vi "validate.vi"(8 "error in":errorcluster, 11 "Shared Memory configuration in":refnum<class "Shared Memory configuration.lvclass">) -> (0 "error out":errorcluster, 3 "Shared Memory configuration out":refnum<class "Shared Memory configuration.lvclass">)   [LabVIEW 2013, in "Shared Memory configuration.lvclass"]
doc: "This function performs validation of the configuration. This function should be safe to call at any point and should not rely on anything in the runtime environment."
uses:
  Shared Memory configuration.lvclass
  <vilib>/NI/Tag Bus Module Framework/module configuration/TBM module configuration.lvclass
  Shared Memory configuration.lvclass/Shared Memory configuration.ctl
  <vilib>/NI/Tag Bus/tag/tag descriptor.lvclass/tag descriptor.ctl
  <vilib>/NI/Tag Bus Module Framework/channel/TBM channel.lvclass/TBM channel.ctl
  <vilib>/NI/Tag Bus/tag/read tag name.vi
  <vilib>/NI/Tag Bus/tag/read data type.vi
  <vilib>/NI/Tag Bus Module Framework/channel/Read channel classification.vi
  <vilib>/NI/Tag Bus Module Framework/channel/TBM channel.lvclass
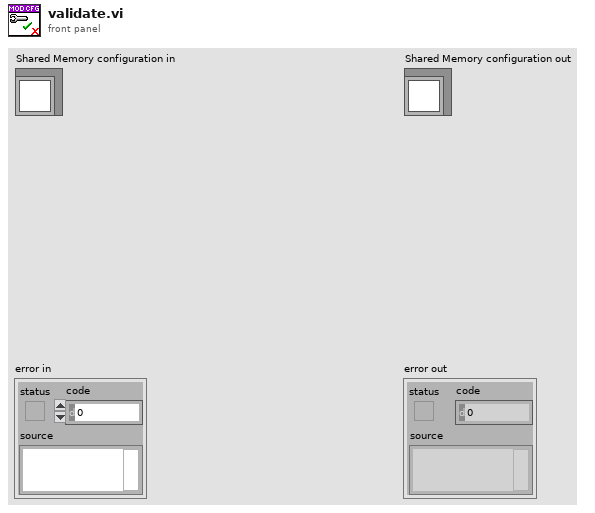
[diagram p1: front panel]
types:
  T1 = typedef "TBM channel.lvclass/channel classification.ctl" = enum16{"input data", "output data", "processing parameter", "processing result"}
  T2 = typedef "tag bus.lvlib/tag descriptor.lvclass/Data Type.ctl" = enum16{"Double", "Single", "I64", "I32", "I16", "I8", "U64", "U32", "U16", "U8", "Boolean", "String", "Array of Double", "Array of Single", "Array of I64", "Array of I32", "Array of I16", "Array of I8", "Array of U64", "Array of U32", "Array of U16", "Array of U8", "Array of Boolean", "Array of String"}
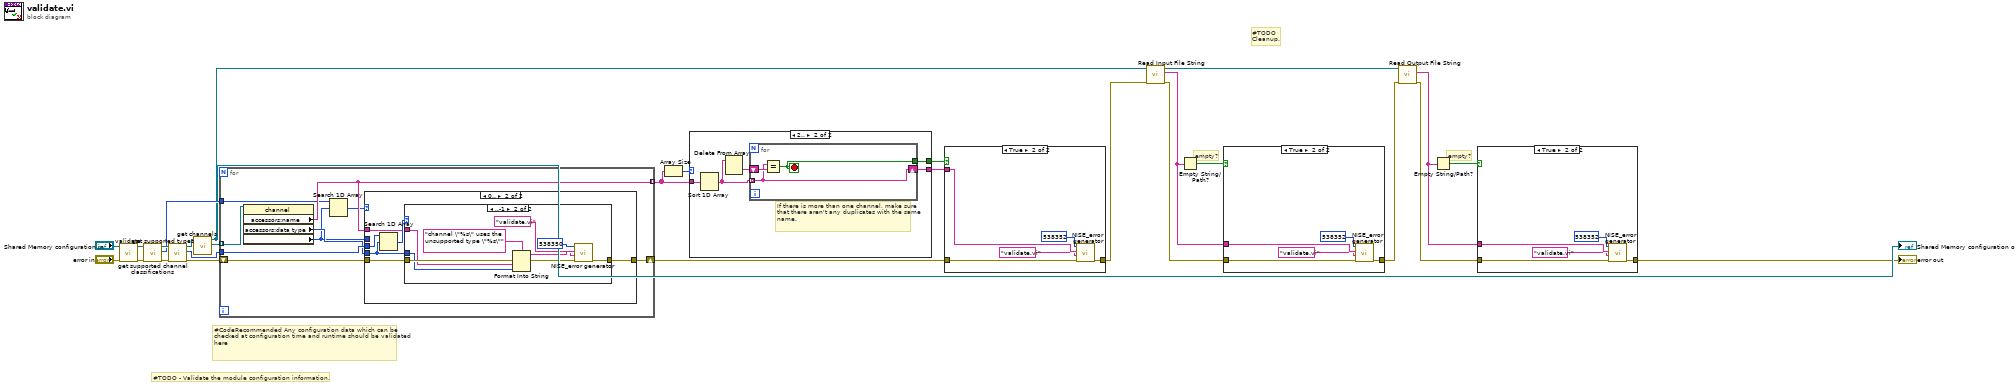
[diagram p0: block diagram]
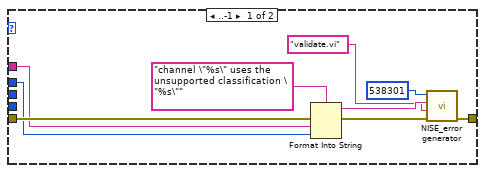
[diagram p6: hidden frame]
diagram:
  # "#TODO\nCleanup."
  # "empty?"
  # "empty?"
  # "#TODO - Validate the module configuration information."
  # "#CodeRecommended Any configuration data which can be checked at configuration time and runtime should be validated here"
  n1 = call-parent "validate.vi"("error in"="error in", "configuration in"="Shared Memory configuration in") -> ("error out"=w27:errorcluster, "configuration out"=w18:refnum<class "Shared Memory configuration.lvclass">)  [unwired: 8 in]
  n2 = call-dynamic "get supported channel classifications.vi"("error in"=w27, "module configuration in"=w18) -> ("error out"=w19:errorcluster, "supported classes"=w16:T1[], "module configuration out"=w17:refnum<class "Shared Memory configuration.lvclass">)  [unwired: 7 in]
  n3 = call-dynamic "get supported types.vi"("error in"=w19, "Shared Memory configuration in"=w17) -> ("error out"=w23:errorcluster, "supported types"=w24:T2[], "Shared Memory configuration out"=w26:refnum<class "Shared Memory configuration.lvclass">)  [unwired: 7 in]
  n4 = call-dynamic "get channels.vi"("Shared Memory configuration in"=w26) -> ("channels"=w25:refnum<class "TBM channel.lvclass">[], "Shared Memory configuration out"=w5:refnum<class "Shared Memory configuration.lvclass">)  [unwired: 9 in]
  "Shared Memory configuration out" <- w5
  n5 = for {
    tunnel: w25 -> [w36] mode=indexing
    tunnel: w24 -> [w35]
    shift-right: [w33] -> w14
    shift-left: w23 -> [w34]
    tunnel: [w31] -> w21 mode=indexing
    tunnel: w16 -> [w30]
    n6 = property class="channel"(reference=w36) -> ("accessors:name"=w31:string, "accessors:data type"=w32:T2, "data access:channel classification"=w28:T1)  [unwired: 1 in, 2 out]
    n7 = Search 1D Array(1D array=w30, element=w28) -> (index of element=w29:i32)  [unwired: 1 in]
    n8 = case shown="0.." w29 {
      tunnel: w35 -> [_ w51]
      tunnel: w34 -> [w41 w49]
      tunnel: [w40 w48] -> w33
      tunnel: w32 -> [_ w47]
      tunnel: w31 -> [w37 w46]
      tunnel: w28 -> [w38 _]
      frame ..-1 {
        n9 = Format Into String(format string="channel \"%s\" uses the unsupported classification \"%s\"", error in=w41, w37, w38) -> (resulting string=w43:string, error out=w44:errorcluster)  [unwired: 1 in]
        n10 = call <vilib>:"NISE_error generator.vi"("error in"=w44, "source"="validate.vi" ("format string"), "append error message"=w43, "error code (0)"=538301) -> ("error out"=w40:errorcluster)  [unwired: 5 in]
      }
      frame 0.. {
        n11 = Search 1D Array(1D array=w51, element=w47) -> (index of element=w50:i32)  [unwired: 1 in]
        n12 = case shown="..-1" w50 {
          tunnel: w49 -> [w52 w56]
          tunnel: [w52 w55] -> w48
          tunnel: w47 -> [_ w54]
          tunnel: w46 -> [_ w53]
          frame 0.. {
          }
          frame ..-1 {
            n13 = Format Into String(format string="channel \"%s\" uses the unsupported type \"%s\"", error in=w56, w53, w54) -> (resulting string=w59:string, error out=w60:errorcluster)  [unwired: 1 in]
            n14 = call <vilib>:"NISE_error generator.vi"("error in"=w60, "source"="validate.vi" ("format string"), "append error message"=w59, "error code (0)"=538350) -> ("error out"=w55:errorcluster)  [unwired: 5 in]
          }
        }
      }
    }
  }
  n15 = Array Size(array=w21) -> (size(s)=w20:i32)
  n16 = case shown="2.." w20 {
    tunnel: [_ w64] -> w13
    tunnel: [_ w63] -> w22
    tunnel: w21 -> [_ w62]
    frame ..1 {
    }
    frame 2.. {
      # "If there is more than one channel, make sure that there aren't any duplicates with the same name."
      n17 = Sort 1D Array(array=w62) -> (sorted array=w65:string[])
      n18 = Delete From Array(array=w65) -> (deleted portion=w66:string)  [unwired: 2 in, 1 out]
      n19 = for {
        shift-right: [w68] -> w63
        shift-left: w66 -> [w69]
        tunnel: w65 -> [w68] mode=indexing
        tunnel: [w67] -> w64
        stop <- w67 stop-if-true
        n20 = Equal?(x=w68, y=w69) -> (x = y?=w67:bool)
      }
    }
  }
  n21 = case shown="True" w13 {
    tunnel: w14 -> [w70 w74]
    tunnel: [w70 w75] -> w4
    tunnel: w22 -> [_ w73]
    frame False {
    }
    frame True {
      n22 = call <vilib>:"NISE_error generator.vi"("error in"=w74, "source"="validate.vi" ("format string"), "append error message"=w73, "error code (0)"=538352) -> ("error out"=w75:errorcluster)  [unwired: 5 in]
    }
  }
  n23 = call "Read Input File String.vi"("error in"=w4, "Shared Memory configuration in"=w5) -> ("error out"=w11:errorcluster, "input file string"=w12:string, "Shared Memory configuration out"=w15:refnum<class "Shared Memory configuration.lvclass">)  [unwired: 7 in]
  n24 = Empty String/Path?(string/path=w12) -> (empty?=w3:bool)
  n25 = case shown="True" w3 {
    tunnel: w11 -> [w76 w80]
    tunnel: [w76 w81] -> w10
    tunnel: w12 -> [_ w79]
    frame False {
    }
    frame True {
      n26 = call <vilib>:"NISE_error generator.vi"("error in"=w80, "source"="validate.vi" ("format string"), "append error message"=w79, "error code (0)"=538352) -> ("error out"=w81:errorcluster)  [unwired: 5 in]
    }
  }
  n27 = call "Read Output File String.vi"("error in"=w10, "Shared Memory configuration in"=w15) -> ("error out"=w9:errorcluster, "output file string"=w8:string)  [unwired: 7 in, 1 out]
  n28 = Empty String/Path?(string/path=w8) -> (empty?=w2:bool)
  n29 = case shown="True" w2 {
    tunnel: w9 -> [w82 w86]
    tunnel: [w82 w87] -> w1
    tunnel: w8 -> [_ w85]
    frame False {
    }
    frame True {
      n30 = call <vilib>:"NISE_error generator.vi"("error in"=w86, "source"="validate.vi" ("format string"), "append error message"=w85, "error code (0)"=538352) -> ("error out"=w87:errorcluster)  [unwired: 5 in]
    }
  }
  "error out" <- w1
